vi "Complex Vector x A (Optimized).vi"(2 "Matrix A":T1, 3 "Vector V'":cdb[](array[numeric])) -> (0 "error":i32, 1 "V' x A":cdb[](array[numeric]))   [LabVIEW 2020, in "NI_AALBase.lvlib"]
uses:
  NI_AALBase.lvlib
  ComplexMatrix.ctl
  <resource>/lvanlys.dll
  NI_Matrix.lvlib
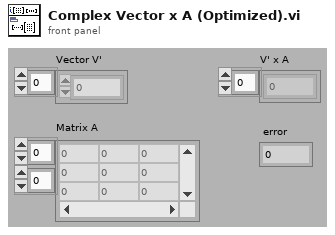
[diagram p1: front panel]
types:
  T1 = typedef "NI_Matrix.lvlib/ComplexMatrix.ctl" = cdb[][]
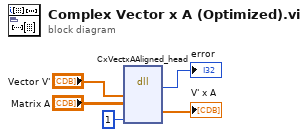
[diagram p0: block diagram]
diagram:
  n1 = dll-call lib="C:/Program Files (x86)/National Instruments/LabVIEW 2020/resource/lvanlys.*" fn="CxVectxAAligned_head"("xHandle"="Vector V'", "aHandle"="Matrix A", "isAligned"=1) -> ("return type"=→"error":i32, "V' x A"=→"V' x A":cdb[])  [unwired: 7 in, 2 out]
